vi "ellie_test.vi"() -> ()   [LabVIEW 2009]
uses:
  <vilib>/express/express signal manip/GetorSetDDTAttributes/Set DDT Attributes/Set DDT Properties.xnode
  <vilib>/express/express shared/transition.llb/Waveform Array To Dynamic.vi
  <vilib>/express/express signal manip/GetorSetDDTAttributes/Set DDT Attributes/SetT0.vi
  <vilib>/express/express shared/transition.llb/Dynamic To Waveform Array.vi
panel:
  in  "Seconds between \nMeasurements":dbl=30.0 min=0.0 max=9999999.0 step=1.0
  out "All Clear":bool
  out "Error":bool
  out "Run Start Time":string
  out "Last Measurement Taken":string
  out "Most Recent Error":string
  out "Heartbeat":bool
  in  "Heartbeat":bool
  in  "Temp Strip Chart":bool
  out "iTC Temperature Strip Chart":dynamicdata(graph)
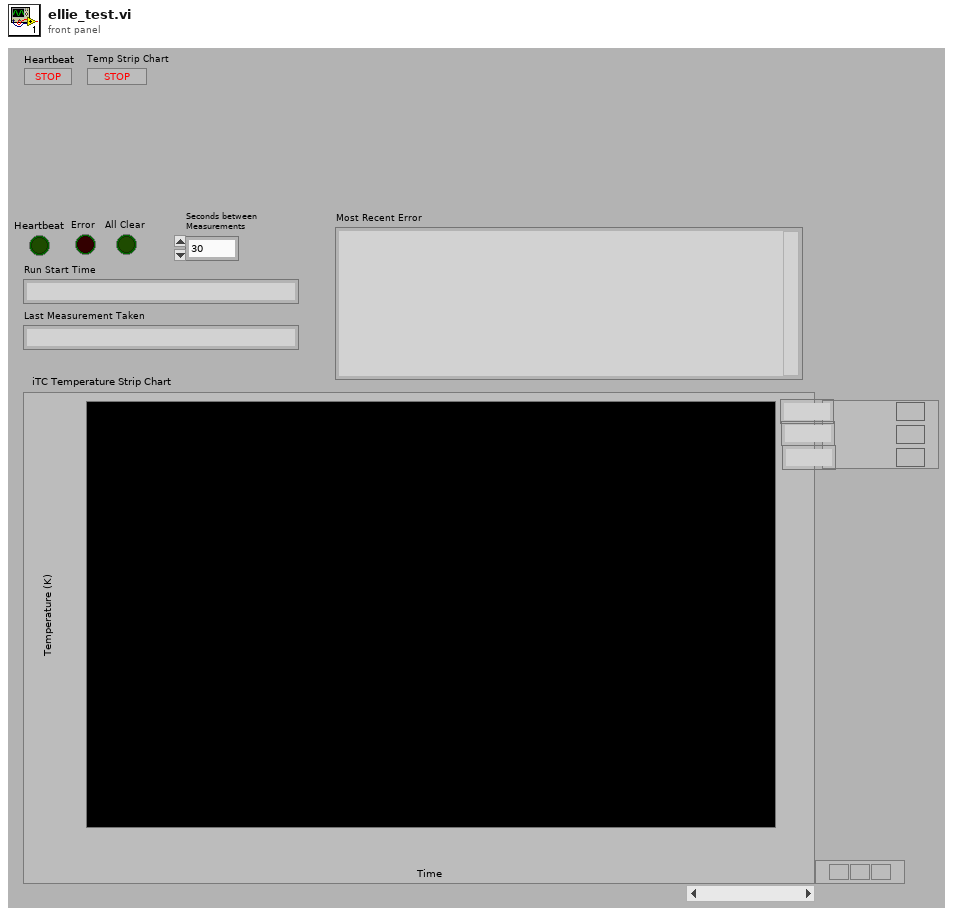
[diagram p1: front panel]
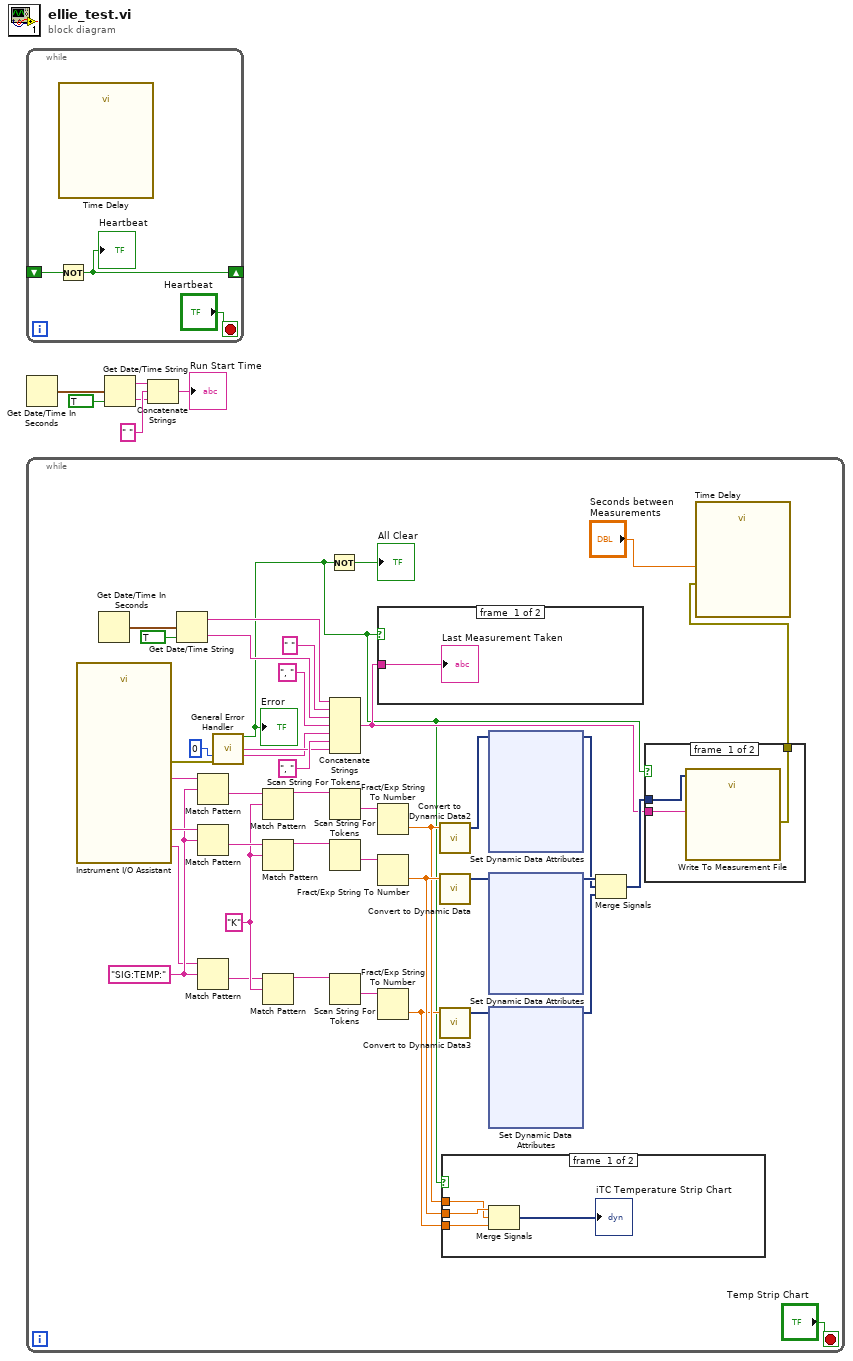
[diagram p0: block diagram]
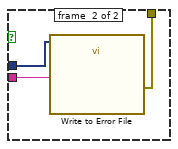
[diagram p3: hidden frame]
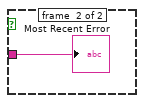
[diagram p4: hidden frame]
diagram:
  n1 = while {
    shift-right: [w7] -> _
    shift-left: _ -> [w9]
    stop <- "Heartbeat" stop-if-true
    n2 = Not(x=w9) -> (.not. x?=w7:bool)
    "Heartbeat" <- w7
    n3 = call "Time Delay"() -> ()  [unwired: 11 in, 1 out]
  }
  n4 = Get Date/Time In Seconds() -> (seconds since 1Jan1904=w5:timestamp)
  n5 = while {
    stop <- "Temp Strip Chart" stop-if-true
    w16 = "SIG:TEMP:"
    w15 = "K"
    n6 = call "Instrument I/O Assistant"() -> ("AB.T"=w14:string, "CCS.T"=w19:string, "Cernox.T"=w22:string, "error out"=w26:errorcluster)  [unwired: 23 in, 1 out]
    n7 = Get Date/Time In Seconds() -> (seconds since 1Jan1904=w46:timestamp)
    n8 = Get Date/Time String(seconds (now)=w46, want seconds? (F)=TRUE) -> (date string=w44:string, time string=w42:string)  [unwired: 1 in]
    n9 = Match Pattern(string=w19, regular expression=w16) -> (after substring=w18:string)  [unwired: 1 in, 3 out]
    n10 = Match Pattern(string=w22, regular expression=w16) -> (after substring=w21:string)  [unwired: 1 in, 3 out]
    n11 = Match Pattern(string=w14, regular expression=w16) -> (after substring=w13:string)  [unwired: 1 in, 3 out]
    n12 = call <vilib>:"General Error Handler.vi"("type of dialog (OK msg:1)"=0, "error in (no error)"=w26) -> ("error?"=w24:bool, "source out"=w30:string, "message"=w29:string)  [unwired: 9 in, 2 out]
    "Error" <- w24
    n13 = Match Pattern(string=w18, regular expression=w15) -> (before substring=w17:string)  [unwired: 1 in, 3 out]
    n14 = Match Pattern(string=w21, regular expression=w15) -> (before substring=w20:string)  [unwired: 1 in, 3 out]
    n15 = Match Pattern(string=w13, regular expression=w15) -> (before substring=w12:string)  [unwired: 1 in, 3 out]
    n16 = Not(x=w24) -> (.not. x?=→"All Clear":bool)
    n17 = Concatenate Strings(w44, " ", w42, ", ", w29, ", ", w30) -> (w27:string)
    n18 = Scan String For Tokens(9:w17) -> (1:w48:string)  [unwired: 5 in, 3 out]
    n19 = Scan String For Tokens(9:w20) -> (1:w50:string)  [unwired: 5 in, 3 out]
    n20 = Scan String For Tokens(9:w12) -> (1:w47:string)  [unwired: 5 in, 3 out]
    n21 = case shown="False" w24 {
      tunnel: w27 -> [w115 w116]
      frame #0 {
        "Last Measurement Taken" <- w115
      }
      frame #1 {
        "Most Recent Error" <- w116
      }
    }
    n22 = Fract/Exp String To Number(string=w48) -> (number=w32:dbl)  [unwired: 3 in, 1 out]
    n23 = Fract/Exp String To Number(string=w50) -> (number=w33:dbl)  [unwired: 3 in, 1 out]
    n24 = Fract/Exp String To Number(string=w47) -> (number=w31:dbl)  [unwired: 3 in, 1 out]
    n25 = call "Convert to Dynamic Data2"("Double"=w32) -> ("Dynamic Data Type"=w37:dynamicdata)  [unwired: 3 in]
    n26 = call "Convert to Dynamic Data"("Double"=w33) -> ("Dynamic Data Type"=w39:dynamicdata)  [unwired: 3 in]
    n27 = call "Convert to Dynamic Data3"("Double"=w31) -> ("Dynamic Data Type"=w36:dynamicdata)  [unwired: 3 in]
    n28 = case shown="False" w24 {
      tunnel: w33 -> [w53 _]
      tunnel: w32 -> [w52 _]
      tunnel: w31 -> [w51 _]
      frame #0 {
        n29 = Merge Signals(w53, w52, w51) -> (→"iTC Temperature Strip Chart":dynamicdata)
      }
      frame #1 {
      }
    }
    n30 = xnode "Set Dynamic Data Attributes"("Signals In"=w37) -> ("Signals Out"=w35:dynamicdata)  [unwired: 4 in, 1 out]
    n31 = xnode "Set Dynamic Data Attributes"("Signals In"=w39) -> ("Signals Out"=w38:dynamicdata)  [unwired: 4 in, 1 out]
    n32 = xnode "Set Dynamic Data Attributes"("Signals In"=w36) -> ("Signals Out"=w34:dynamicdata)  [unwired: 4 in, 1 out]
    n33 = Merge Signals(w38, w35, w34) -> (w28:dynamicdata)
    n34 = case shown="False" w24 {
      tunnel: w28 -> [w57 w60]
      tunnel: w27 -> [w56 w59]
      tunnel: [w55 w58] -> w11
      frame #0 {
        n35 = call "Write To Measurement File"("Signals"=w57, "Comment"=w56) -> ("error out"=w55:errorcluster)  [unwired: 15 in, 2 out]
      }
      frame #1 {
        n36 = call "Write to Error File"("Signals"=w60, "Comment"=w59) -> ("error out"=w58:errorcluster)  [unwired: 15 in, 2 out]
      }
    }
    n37 = call "Time Delay"("error in (no error)"=w11, "Delay Time (s)"="Seconds between \nMeasurements") -> ()  [unwired: 9 in, 1 out]
  }
  n38 = Get Date/Time String(seconds (now)=w5, want seconds? (F)=TRUE) -> (date string=w4:string, time string=w2:string)  [unwired: 1 in]
  n39 = Concatenate Strings(w4, " ", w2) -> (→"Run Start Time":string)
